vi "AppData - Set.vi"(4 "error in":errorcluster, 7 "Data In":T1 {"LogStartTime" format="%<%x %.3X>T"}) -> (0 "error out":errorcluster, 3 "Data Out":T1 {"LogStartTime" format="%<%x %.3X>T"})   [LabVIEW 2023]
uses:
  controls/UI Data.ctl
  <vilib>/NI/Modbus Library/API/Master/Modbus Master.lvclass
  LibreVNA/LibreVNA.lvclass
  controls/Action Enum.ctl
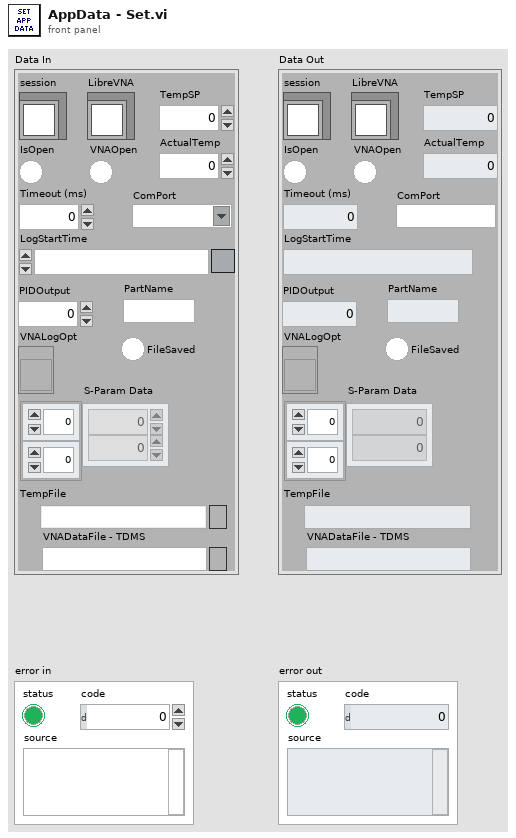
[diagram p1: front panel]
types:
  T1 = typedef "UI Data.ctl" = cluster{"session":refnum<class "Modbus Master.lvclass">, "IsOpen":bool, "Timeout (ms)":i32, "TempFile":path, "LogStartTime":timestamp, "LibreVNA":refnum<class "LibreVNA.lvclass">, "VNAOpen":bool, "TempSP":dbl, "ActualTemp":dbl, "FileSaved":bool, "PIDOutput":dbl, "VNALogOpt":refnum<vi>, "PartName":string, "ComPort":refnum<visa-resource-name>, "S-Param Data":dbl[][], "VNADataFile - TDMS":path}
  T2 = typedef "Action Enum.ctl" = enum16{"GET", "SET", "RESET"}
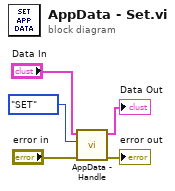
[diagram p0: block diagram]
diagram:
  n1 = call "AppData - Handle.vi"("error in"="error in", "Action"=Action_Enum."SET", "Data In"="Data In") -> ("error out"=→"error out":errorcluster, "Data Out"=→"Data Out":T1)  [unwired: 3 in]
